vi "Digitizer Scan Fetch Last.vi"(7 "ValBufferSize":i32=2048, 8 "error in (no error)":errorcluster {"code" format="%.0x"}, 9 "Channel":i32, 10 "Count":i32 format="%.0g", 11 "instrument handle":refnum<k15>) -> (0 "error out":errorcluster {"code" format="%.0x"}, 1 "ValActualSize":i32, 2 "Val":dbl[](array[numeric]) format="%.2p", 3 "instrument handle out":refnum<k15>)   [LabVIEW 2020, in "Keysight DAQ970.lvlib"]
doc: "Returns the most recent reading(s) in the last record on the specified channel."
uses:
  Keysight DAQ970.lvlib
  KtDAQ970.dll
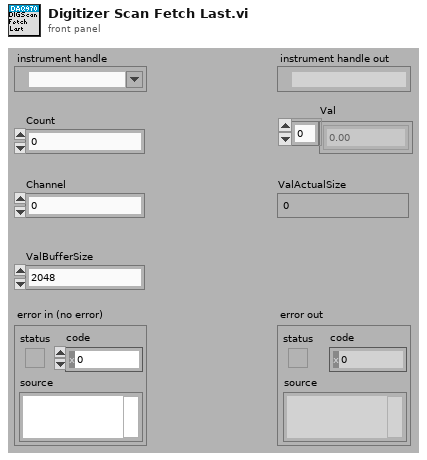
[diagram p1: front panel]
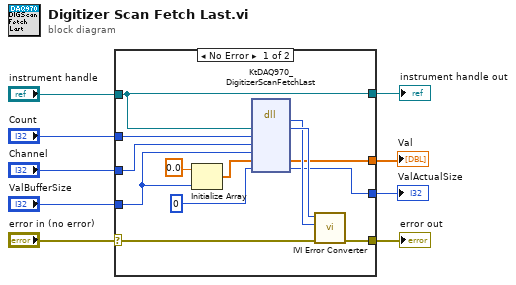
[diagram p0: block diagram]
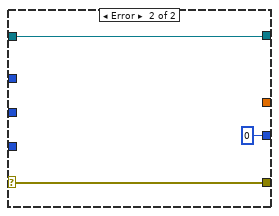
[diagram p2: hidden frame]
diagram:
  n1 = case shown="No Error" "error in (no error)" {
    selector: "error in (no error)" -> [w20 w25]
    tunnel: [w19 w25] -> w9
    tunnel: "instrument handle" -> [w15 w24]
    tunnel: "Count" -> [w18 _]
    tunnel: "Channel" -> [w17 _]
    tunnel: "ValBufferSize" -> [w13 _]
    tunnel: [w16 _] -> w2
    tunnel: [w15 w24] -> w3
    tunnel: [w10 0 ("ValActualSize")] -> w1
    frame No Error {
      n2 = Initialize Array(0.0 ("element"), w13) -> (w12:dbl[])
      n3 = dll-call lib="KtDAQ970**.dll" fn="KtDAQ970_DigitizerScanFetchLast"("Vi"=w15, "Count"=w18, "Channel"=w17, "ValBufferSize"=w13, "Val"=w12, "ValActualSize"=0) -> ("return type"=w21:i32, "Vi"=w22:u32, "Val"=w16:dbl[], "ValActualSize"=w10:i32)  [unwired: 6 in, 2 out]
      n4 = call "IVI Error Converter.vi"("error in (no error)"=w20, "IVI error code (0)"=w21, "instrument handle"=w22) -> ("error out"=w19:errorcluster)  [unwired: 7 in, 1 out]
    }
    frame Error {
    }
  }
  "error out" <- w9
  "instrument handle out" <- w3
  "Val" <- w2
  "ValActualSize" <- w1
